vi "Source Limit Power.vi"(0 "VISA resource name":refnum<visa-resource-name>, 5 "Node In":string, 7 "Channel (Channel A)":u16(ring) items=["Channel A", "Channel B"], 9 "Power limit (watts)":sgl, 11 "error in (no error)":errorcluster) -> (4 "VISA resource name out":refnum<visa-resource-name>, 6 "Node Out":string, 15 "error out":errorcluster)   [LabVIEW 2013, in "Keithley 2600 Series.lvlib"]
doc: "This VI controls the power compliance limit.\n\n<b>Functions and Attributes Used</b>\nsmux.source.limitp"
uses:
  Keithley 2600 Series.lvlib
  Private/GlobalVariables.vi
panel:
  # "(c) 2010 Keithley Instruments, Inc.  ALL RIGHTS RESERVED."
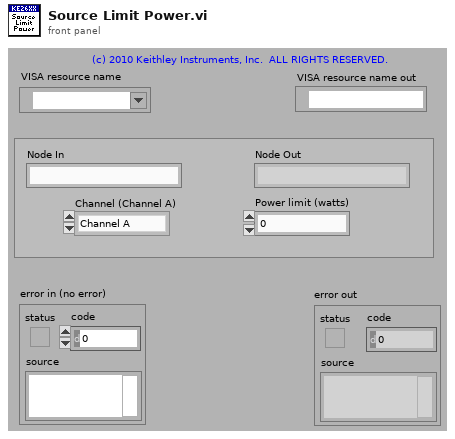
[diagram p1: front panel]
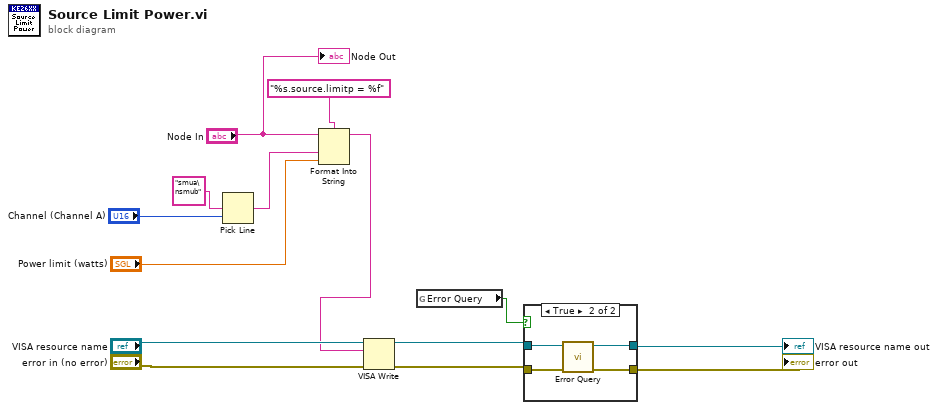
[diagram p0: block diagram]
diagram:
  n1 = Pick Line(multi-line string="smua\nsmub", line index="Channel (Channel A)") -> (output string=w5:string)  [unwired: 1 in]
  n2 = Format Into String(format string="%s.source.limitp = %f", initial string="Node In", w5, "Power limit (watts)") -> (resulting string=w3:string)  [unwired: 1 in, 1 out]
  n3 = VISA Write(VISA resource name="VISA resource name", write buffer=w3, error in (no error)="error in (no error)") -> (VISA resource name out=w13:refnum<visa-resource-name>, error out=w12:errorcluster)  [unwired: 1 out]
  n4 = global read "GlobalVariables.vi" "Error Query"() -> (w14:bool)
  n5 = case shown="True" w14 {
    tunnel: w13 -> [w16 w20]
    tunnel: w12 -> [w15 w19]
    tunnel: [w16 w18] -> w2
    tunnel: [w15 w17] -> w1
    frame False {
    }
    frame True {
      n6 = call "Error Query.vi"("error in (no error)"=w19, "VISA resource name"=w20) -> ("error out"=w17:errorcluster, "VISA resource name out"=w18:refnum<visa-resource-name>)  [unwired: 8 out]
    }
  }
  "VISA resource name out" <- w2
  "error out" <- w1
  "Node Out" <- "Node In"
